vi "Init.vi"(8 "error in (no error)":errorcluster, 9 "Port":u16=4663, 10 "Run External":bool, 11 "Control VI":T1) -> (0 "error out":errorcluster, 3 "FormulaLV App out":refnum<class "FormulaG App.lvclass">)   [LabVIEW 2024, in "FormulaG.lvlib" / "FormulaG App.lvclass"]
uses:
  FormulaG App.lvclass
  FormulaG-Common/Control VI.ctl
  State Update.ctl
  FormulaG-Common/Car State.ctl
  FormulaG-Common/Ranges.ctl
  FormulaG-Common/Car Info.ctl
  FormulaG-Common/Car Control.ctl
  Command/Command.lvclass
  FormulaG App.lvclass/FormulaG App.ctl
  FormulaG-Common/FormulaG-Common.lvlib
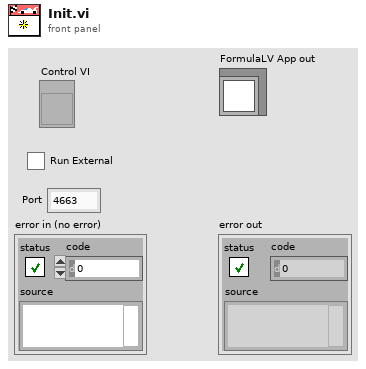
[diagram p1: front panel]
types:
  T1 = typedef "FormulaG-Common.lvlib/Control VI.ctl" = refnum<vi>
  T2 = typedef "FormulaG.lvlib/FormulaG App.lvclass/State Update.ctl" = cluster{"Car State":T3, "Car Control":T6, "Update Rate":dbl, "error":errorcluster}
  T3 = typedef "FormulaG-Common.lvlib/Car State.ctl" = cluster{"Ranges":T4, "Car Info":T5, "Current Lap":dbl, "Last Lap":dbl, "Lap":u8}
  T4 = typedef "FormulaG-Common.lvlib/Ranges.ctl" = cluster{"Front":sgl[], "Rear":sgl[]}
  T5 = typedef "FormulaG-Common.lvlib/Car Info.ctl" = cluster{"Speed":sgl, "X":sgl, "Y":sgl, "Heading":sgl}
  T6 = typedef "FormulaG-Common.lvlib/Car Control.ctl" = cluster{"Steering (-1 to 1)":sgl, "Throttle (0 to 1)":sgl}
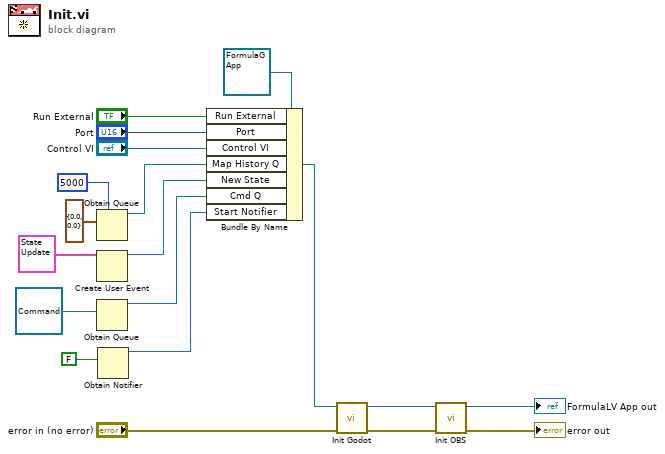
[diagram p0: block diagram]
diagram:
  n1 = Obtain Queue(max queue size (-1, unlimited)=5000, element data type=cluster{dbl, dbl} {0.0, 0.0}) -> (queue out=w13:refnum<queue>)  [unwired: 3 in, 2 out]
  n2 = Create User Event(user event datatype=T2 {"Car State"={"Ranges"={"Front"=[], "Rear"=[]}, "Car Info"={"Speed"=0.0, "X"=0.0, "Y"=0.0, "Heading"=0.0}, "Current Lap"=0.0, "Last Lap"=0.0, "Lap"=0}, "Car Control"={"Steering (-1 to 1)"=0.0, "Throttle (0 to 1)"=0.0}, "Update Rate"=0.0, "error"={"status"=FALSE, "code"=0, "source"=""}} ("State Update")) -> (user event=w11:refnum<user-event>)  [unwired: 1 in, 1 out]
  n3 = Obtain Queue(element data type=refnum<class "Command.lvclass"> refnum ("FormulaG.lvlib:Command.lvclass")) -> (queue out=w7:refnum<queue>)  [unwired: 4 in, 2 out]
  n4 = Obtain Notifier(notification data type=FALSE) -> (notifier out=w1:refnum<notifier>)  [unwired: 3 in, 2 out]
  n5 = Bundle By Name(cluster=refnum<class "FormulaG App.lvclass"> refnum ("FormulaLV App in"), "Run External"="Run External", "Port"="Port", "Control VI"="Control VI", "Map History Q"=w13, "New State"=w11, "Cmd Q"=w7, "Start Notifier"=w1) -> (w17:refnum<class "FormulaG App.lvclass">)
  n6 = call "Init Godot.vi"("error in (no error)"="error in (no error)", "FormulaLV App in"=w17) -> ("error out"=w19:errorcluster, "FormulaLV App out"=w4:refnum<class "FormulaG App.lvclass">)  [unwired: 8 in]
  n7 = call "Init OBS.vi"("error in (no error)"=w19, "FormulaG App in"=w4) -> ("error out"=→"error out":errorcluster, "FormulaG App out"=→"FormulaLV App out":refnum<class "FormulaG App.lvclass">)  [unwired: 8 in]
